vi "WindowBuild_2.vi"(7 "Init":bool, 8 "Error In":errorcluster, 11 "Fitter in":refnum<class "FitterBase.lvclass">=refnum) -> (0 "Error Out":errorcluster, 2 "Timeout":bool, 3 "Fitter out":refnum<class "FitterBase.lvclass">)   [LabVIEW 2018, in "AnalysisPlugins.lvlib" / "FitterBase.lvclass"]
uses:
  FitterBase.lvclass
  C:/projects/ICDAS/NistPluggableModules/Analysis/AnalysisPlugins/AnalysisPluginBaseClass/AnalysisPluginsBase.lvclass
  PmuAnalysisClass/PmuAnalysis.lvclass
  FGen/MemberClasses/PmuTestFunctions/PmuTestFunctions.lvclass
  AnalysisPluginBaseClass/Typedefs/SampleDataInput.ctl
  AnalysisPluginBaseClass/AnalysisPluginsBase.lvclass/AnalysisPluginsBase.ctl
  Typedefs/Wvfrm_ref.ctl
  AnalysisPluginBaseClass/Accessors/Read Window.vi
  AnalysisPluginBaseClass/Accessors/Read SensorQue.vi
  AnalysisPluginBaseClass/Accessors/Read Duration.vi
  AnalysisPluginBaseClass/Accessors/Read AnalysisTime.vi
  AnalysisPluginBaseClass/Accessors/Read SampleDataQueName.vi
  AnalysisPluginBaseClass/Accessors/Write Window.vi
  <vilib>/Utility/error.llb/Error Cluster From Error Code.vi
  <vilib>/ErrorRing/Error Ring.xnode
  AnalysisPluginBaseClass/AnalysisPluginsBase.lvclass
panel:
  out "SampleData":dbl[][](graph)
  out "Window":dbl[][](graph)
  out "T0":timestamp format="%^<%.3X\n%x>T"
  out "SensorTime":timestamp format="%^<%.3X\n%x>T"
  out "WindowTime":timestamp format="%^<%.3X\n%x>T"
  out "SampleTime":timestamp format="%^<%.3X\n%x>T"
  out "Continue":bool
  out "Valid":bool
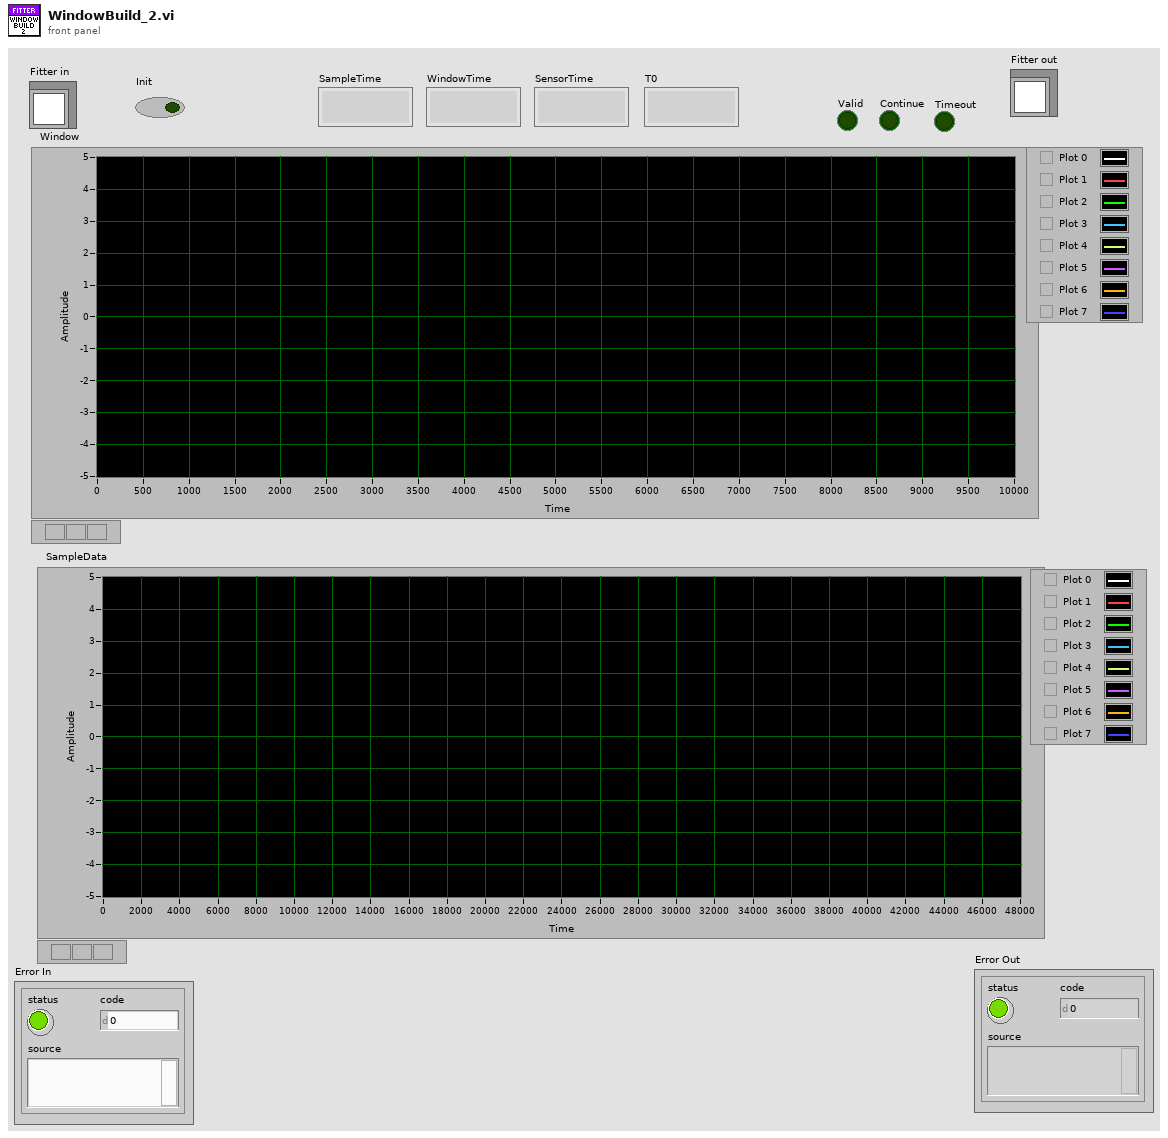
[diagram p1: front panel]
types:
  T1 = typedef "AnalysisPlugins.lvlib/AnalysisPluginsBase.lvclass/SampleDataInput.ctl" = waveform(dbl)[]
  T2 = typedef "AnalysisPlugins.lvlib/FitterBase.lvclass/Wvfrm_ref.ctl" = cluster{"t0":timestamp, "dt":dbl, "attributes":variant, "Y_ref":refnum<data-value>}
  T3 = typedef "AnalysisPlugins.lvlib/AnalysisPluginsBase.lvclass/clWindowData.ctl" = cluster{"Timestamp":ext, "Samples":dbl[][], "Window Valid":bool, "T0":ext}
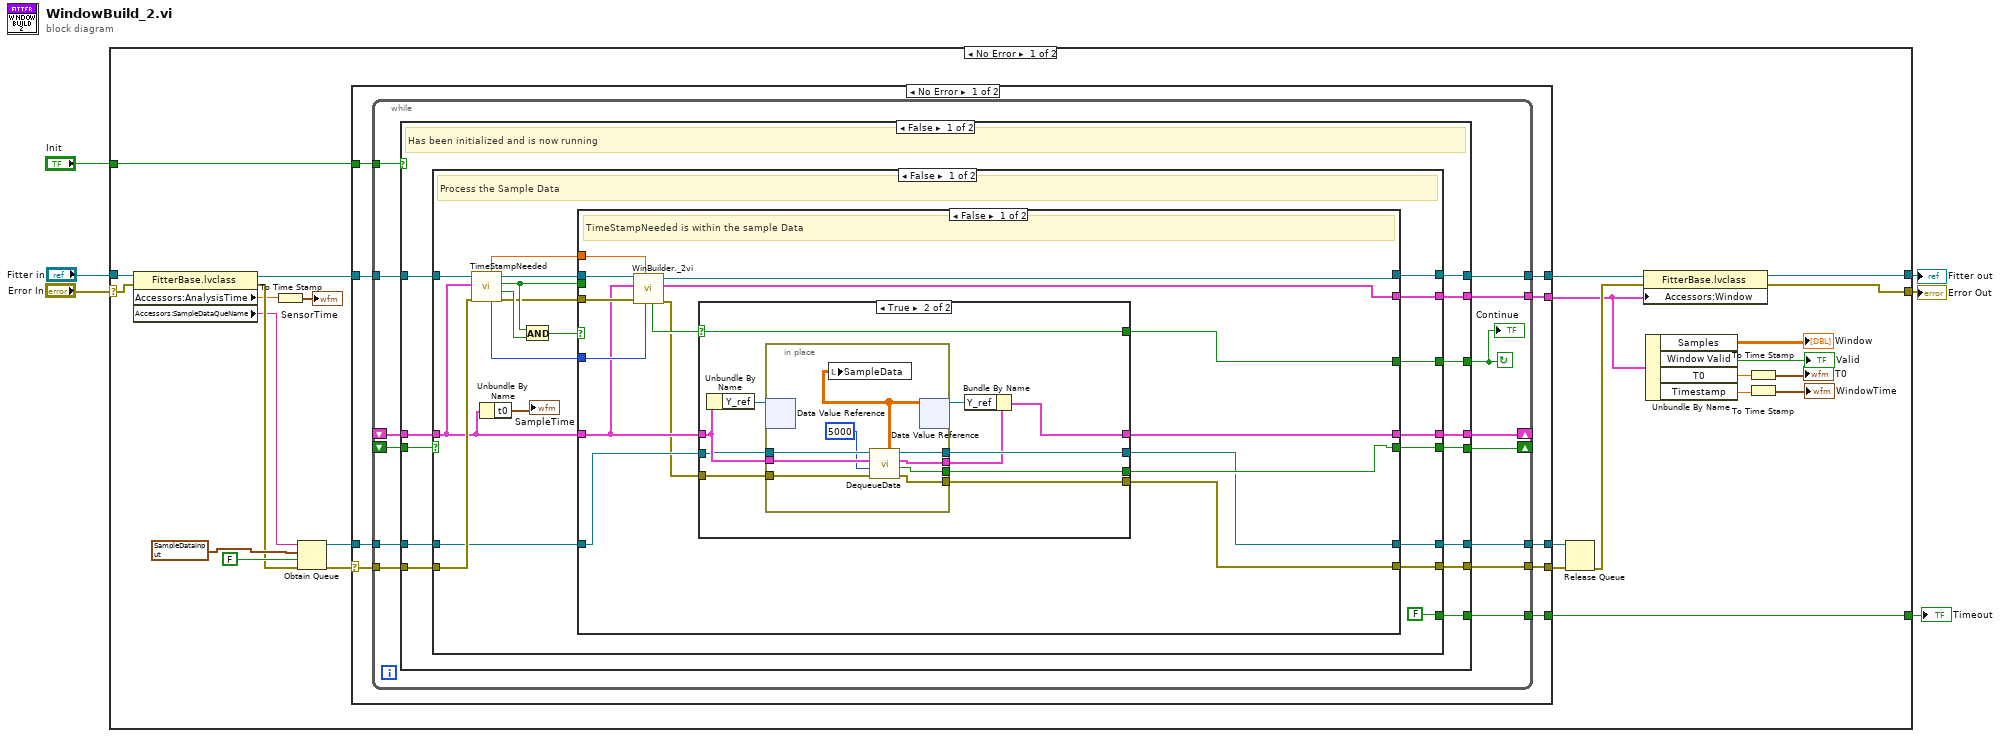
[diagram p0: block diagram]
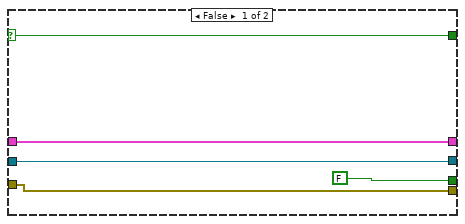
[diagram p2: hidden frame]
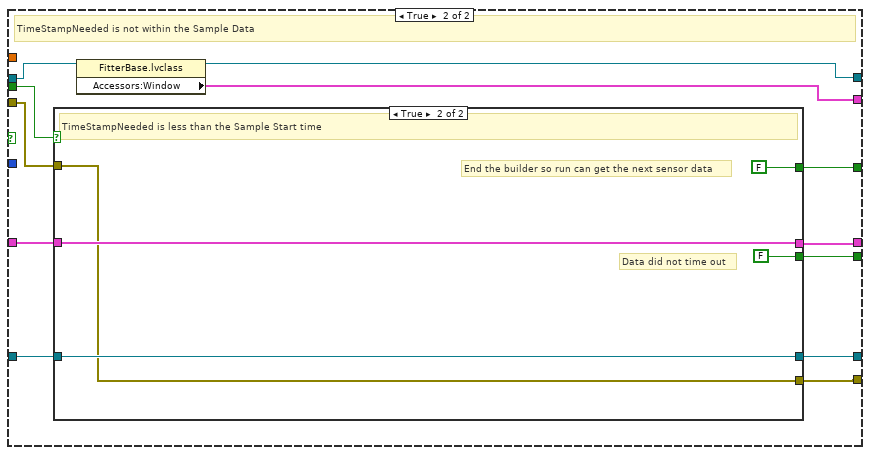
[diagram p3: hidden frame]
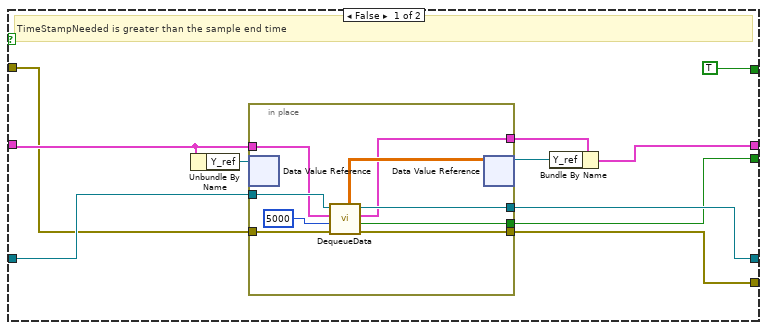
[diagram p4: hidden frame]
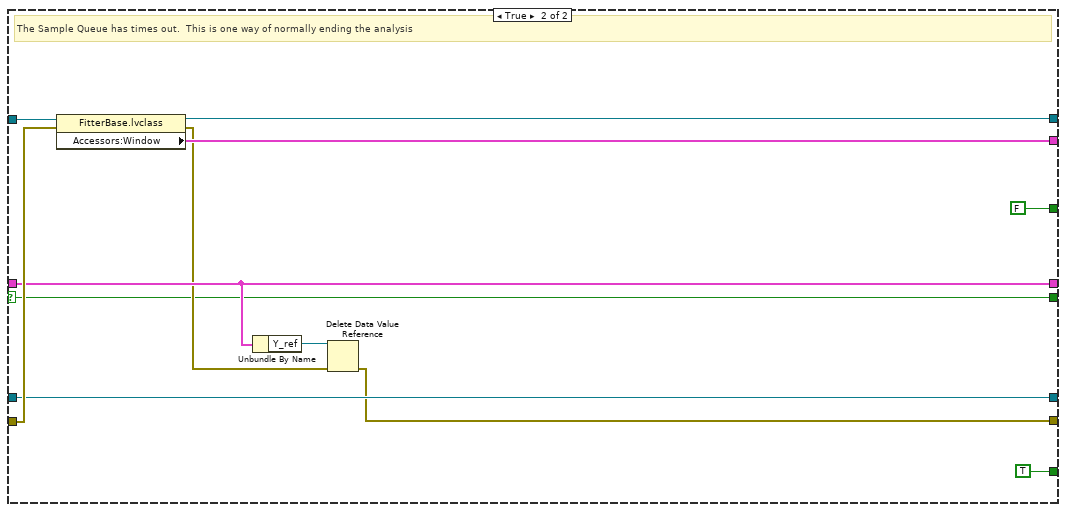
[diagram p5: hidden frame]
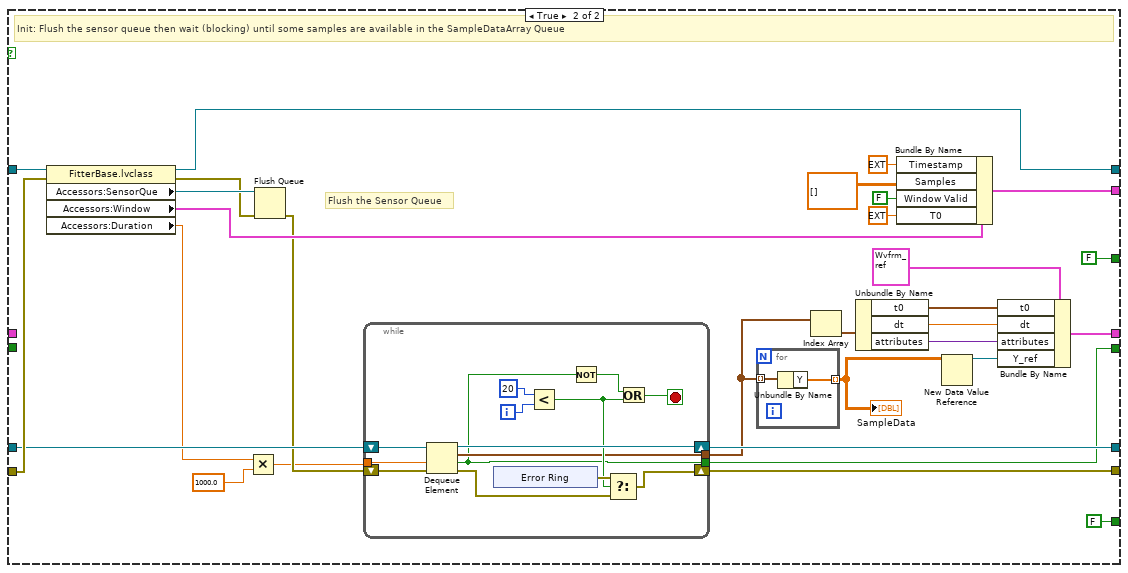
[diagram p6: hidden frame]
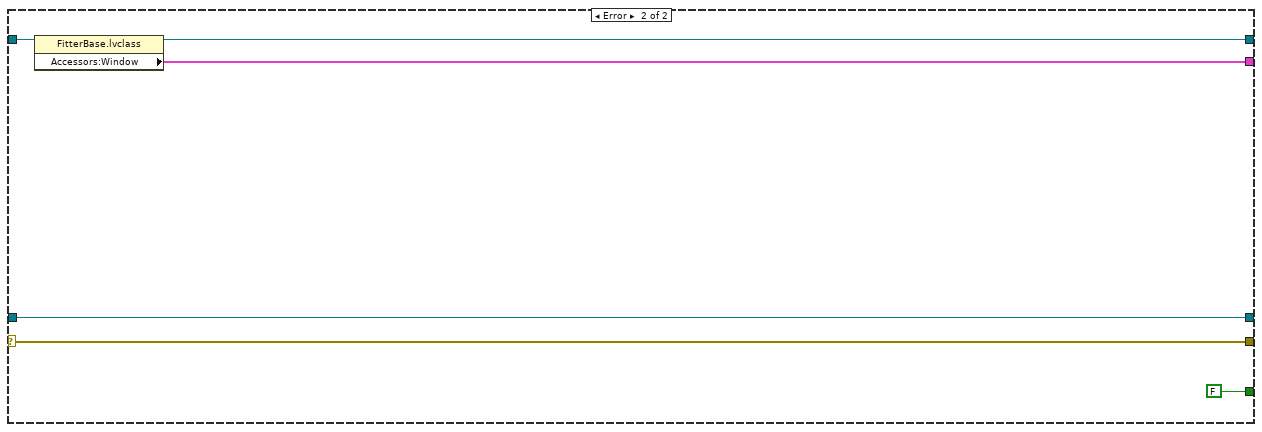
[diagram p7: hidden frame]
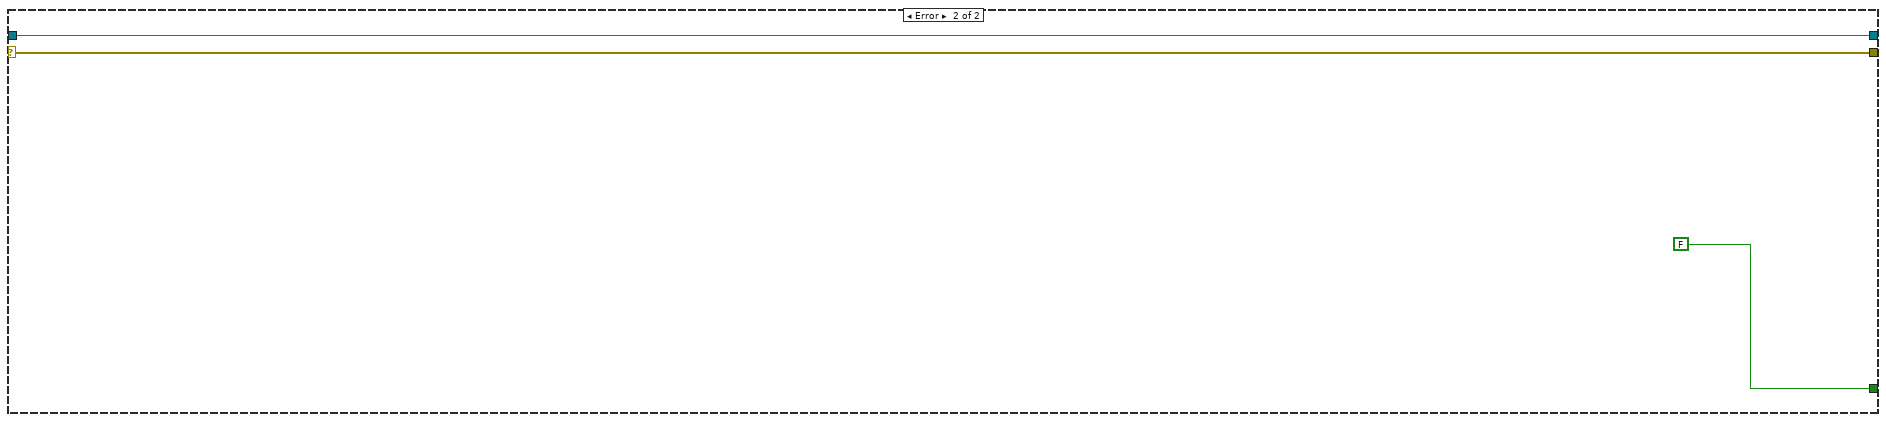
[diagram p8: hidden frame]
diagram:
  n1 = case shown="No Error" "Error In" {
    selector: "Error In" -> [w31 w235]
    tunnel: "Fitter in" -> [w32 w236]
    tunnel: [w18 w236] -> w4
    tunnel: [w17 w235] -> w3
    tunnel: [w19 FALSE] -> w2
    tunnel: "Init" -> [w20 _]
    frame No Error {
      n2 = property class="FitterBase.lvclass"(reference=w32, error in=w31) -> (reference out=w26:refnum<class "FitterBase.lvclass">, error out=w25:errorcluster, "Accessors:AnalysisTime"=w8:dbl, "Accessors:SampleDataQueName"=w9:string)
      n3 = To Time Stamp(1:w8) -> (0:→"SensorTime":timestamp)
      n4 = Obtain Queue(name (unnamed)=w9, element data type=T1 [{"t0"=timestamp(0 s since 1904-01-01), "dt"=1.0, "Y"=[]}] ("clSampleDataArray"), create if not found? (T)=FALSE, error in (no error)=w25) -> (queue out=w27:refnum<queue>, error out=w28:errorcluster)  [unwired: 1 in, 1 out]
      n5 = case shown="No Error" w28 {
        selector: w28 -> [w39 w231]
        tunnel: w27 -> [w37 w232]
        tunnel: [w33 w230] -> w22
        tunnel: w26 -> [w40 w233]
        tunnel: [w36 w232] -> w24
        tunnel: [w35 w231] -> w23
        tunnel: [w38 w229] -> w16
        tunnel: w20 -> [w41 _]
        tunnel: [w34 FALSE] -> w19
        frame No Error {
          n6 = while {
            tunnel: w41 -> [w55]
            tunnel: w40 -> [w54]
            tunnel: w39 -> [w53]
            tunnel: [w52] -> w38
            tunnel: w37 -> [w51]
            tunnel: [w50] -> w36
            tunnel: [w49] -> w35
            shift-right: [w48] -> _
            shift-left: _ -> [w43]
            shift-right: [w47] -> _
            shift-left: _ -> [w44]
            tunnel: [w46] -> w34
            tunnel: [w45] -> w33
            stop <- w42 continue-if-true
            n7 = case shown="False" w55 {
              tunnel: w54 -> [w67 w207]
              tunnel: w53 -> [w66 w206]
              tunnel: [w64 w197] -> w52
              tunnel: w51 -> [w59 w196]
              tunnel: [w58 w192] -> w50
              tunnel: [w57 w191] -> w49
              tunnel: [w62 w182] -> w48
              tunnel: [w56 w181] -> w47
              tunnel: [w60 FALSE] -> w46
              tunnel: [w61 FALSE] -> w42
              tunnel: [w65 w178] -> w45
              tunnel: w44 -> [w68 _]
              tunnel: w43 -> [w63 _]
              frame False {
                # "Has been initialized and is now running"
                n8 = case shown="False" w68 {
                  selector: w68 -> [_ w166]
                  tunnel: w67 -> [w88 w177]
                  tunnel: w66 -> [w87 w176]
                  tunnel: [w74 w175] -> w65
                  tunnel: [w73 w174] -> w64
                  tunnel: w63 -> [w70 w173]
                  tunnel: [w80 w173] -> w62
                  tunnel: [w83 FALSE] -> w61
                  tunnel: [FALSE TRUE] -> w60
                  tunnel: [w78 w168] -> w58
                  tunnel: w59 -> [w82 w168]
                  tunnel: [w79 w167] -> w57
                  tunnel: [w77 w166] -> w56
                  frame False {
                    # "Process the Sample Data"
                    n9 = call "TimeStampNeeded.vi"("Error In"=w87, "Wvfrm_ref"=w70, "Fitter In"=w88) -> ("Error Out"=w81:errorcluster, "TsnGreaterThanSampleStart"=w85:bool, "TsnLessThanSample Start Time"=w84:bool, "Fitter Out"=w76:refnum<class "FitterBase.lvclass">, "nSamplesNeeded"=w72:i32, "TimeStampNeeded"=w75:ext)  [unwired: 3 in]
                    n10 = Unbundle By Name(w70) -> ("t0"=→"SampleTime":timestamp)
                    n11 = And(x=w84, y=w85) -> (x .and. y?=w86:bool)
                    n12 = case shown="False" w86 {
                      tunnel: w84 -> [_ w140]
                      tunnel: [w95 w139] -> w83
                      tunnel: w70 -> [w97 w138]
                      tunnel: w82 -> [w94 w137]
                      tunnel: w81 -> [w102 w136]
                      tunnel: [w89 w135] -> w80
                      tunnel: [w91 w134] -> w79
                      tunnel: [w90 w133] -> w78
                      tunnel: [w92 w132] -> w77
                      tunnel: w76 -> [w103 w131]
                      tunnel: w75 -> [w101 _]
                      tunnel: [w99 w130] -> w74
                      tunnel: [w98 w129] -> w73
                      tunnel: w72 -> [w100 _]
                      frame False {
                        # "TimeStampNeeded is within the sample Data"
                        n13 = call "WinBuilder._2vi.vi"("nSampleNeeded"=w100, "TimeStampNeeded"=w101, "Error In"=w102, "Wvfrm_ref"=w97, "Fitter In"=w103) -> ("Error Out"=w93:errorcluster, "Window"=w98:T3, "Fitter Out"=w99:refnum<class "FitterBase.lvclass">, "Continue"=w96:bool)  [unwired: 2 in, 1 out]
                        n14 = case shown="True" w96 {
                          selector: w96 -> [w105 w113]
                          tunnel: w94 -> [w108 w117]
                          tunnel: w97 -> [w107 w119]
                          tunnel: w93 -> [w106 w116]
                          tunnel: [w108 w115] -> w90
                          tunnel: [w107 w110] -> w89
                          tunnel: [w106 w114] -> w91
                          tunnel: [w105 w113] -> w95
                          tunnel: [FALSE w112] -> w92
                          frame False {
                          }
                          frame True {
                            n15 = Unbundle By Name(w119) -> ("Y_ref"=w118:refnum<data-value>)
                            n16 = in-place {
                              in-place-border: w119 -> [w127]
                              in-place-border: w117 -> [w128]
                              in-place-border: w116 -> [w125]
                              in-place-border: [w124] -> w115
                              in-place-border: [w123] -> w111
                              in-place-border: [w122] -> w112
                              in-place-border: [w121] -> w114
                              n17 = in-place-dvr #1(w118) -> ()  [unwired: 2 out]
                              n18 = call "DequeueData.vi"("error in (no error)"=w125, "timeout in ms (-1)"=5000, "DataIn"=w127, "queue in"=w128) -> ("error out"=w121:errorcluster, "timed out?"=w122:bool, "Data Out"=w123:T2, "queue out"=w124:refnum<queue>, "Y"=w120:dbl[][])  [unwired: 3 in]
                              n19 = local write "SampleData"(w120) -> ()
                              n20 = in-place-dvr #1(w120) -> (w109:refnum<data-value>)  [unwired: 1 out]
                            }
                            n21 = Bundle By Name(cluster=w111, "Y_ref"=w109) -> (w110:T2)
                          }
                        }
                      }
                      frame True {
                        # "TimeStampNeeded is not within the Sample Data"
                        n22 = case shown="True" w140 {
                          tunnel: [TRUE FALSE] -> w139
                          tunnel: w138 -> [w147 w164]
                          tunnel: w137 -> [w146 w162]
                          tunnel: w136 -> [w145 w161]
                          tunnel: [w144 w164] -> w135
                          tunnel: [w143 w161] -> w134
                          tunnel: [w142 w162] -> w133
                          tunnel: [w141 FALSE] -> w132
                          frame False {
                            # "TimeStampNeeded is greater than the sample end time"
                            n23 = Unbundle By Name(w147) -> ("Y_ref"=w148:refnum<data-value>)
                            n24 = in-place {
                              in-place-border: w145 -> [w160]
                              in-place-border: w146 -> [w158]
                              in-place-border: w147 -> [w157]
                              in-place-border: [w156] -> w142
                              in-place-border: [w155] -> w143
                              in-place-border: [w154] -> w141
                              in-place-border: [w152] -> w149
                              n25 = in-place-dvr #2(w148) -> ()  [unwired: 2 out]
                              n26 = call "DequeueData.vi"("error in (no error)"=w160, "timeout in ms (-1)"=5000, "DataIn"=w157, "queue in"=w158) -> ("error out"=w155:errorcluster, "timed out?"=w154:bool, "Data Out"=w152:T2, "queue out"=w156:refnum<queue>, "Y"=w153:dbl[][])  [unwired: 3 in]
                              n27 = in-place-dvr #2(w153) -> (w150:refnum<data-value>)  [unwired: 1 out]
                            }
                            n28 = Bundle By Name(cluster=w149, "Y_ref"=w150) -> (w144:T2)
                          }
                          frame True {
                            # "Data did not time out"
                            # "End the builder so run can get the next sensor data"
                            # "TimeStampNeeded is less than the Sample Start time"
                          }
                        }
                        n29 = property class="FitterBase.lvclass"(reference=w131) -> (reference out=w130:refnum<class "FitterBase.lvclass">, "Accessors:Window"=w129:T3)  [unwired: 1 in, 1 out]
                      }
                    }
                  }
                  frame True {
                    # "The Sample Queue has times out.  This is one way of normally ending the analysis"
                    n30 = property class="FitterBase.lvclass"(reference=w177, error in=w176) -> (reference out=w175:refnum<class "FitterBase.lvclass">, error out=w171:errorcluster, "Accessors:Window"=w174:T3)
                    n31 = Unbundle By Name(w173) -> ("Y_ref"=w172:refnum<data-value>)
                    n32 = Delete Data Value Reference(data value reference=w172, error in=w171) -> (error out=w167:errorcluster)  [unwired: 1 out]
                  }
                }
              }
              frame True {
                # "Flush the Sensor Queue"
                # "Init: Flush the sensor queue then wait (blocking) until some samples are available in the SampleDataArray Queue"
                n33 = property class="FitterBase.lvclass"(reference=w207, error in=w206) -> (reference out=w178:refnum<class "FitterBase.lvclass">, error out=w203:errorcluster, "Accessors:SensorQue"=w204:refnum<queue>, "Accessors:Window"=w202:T3, "Accessors:Duration"=w194:dbl)
                n34 = Multiply(x=w194, y=1000.0) -> (x*y=w193:dbl)
                n35 = Flush Queue(queue=w204, error in (no error)=w203) -> (error out=w195:errorcluster)  [unwired: 2 out]
                n36 = while {
                  shift-right: [w218] -> w192
                  shift-left: w196 -> [w223]
                  shift-right: [w219] -> w191
                  shift-left: w195 -> [w222]
                  tunnel: w193 -> [w213]
                  tunnel: [w211] -> w184
                  tunnel: [w210] -> w181
                  i -> [w215]
                  stop <- w212 stop-if-true
                  n37 = Dequeue Element(queue=w223, timeout in ms (-1)=w213, error in (no error)=w222) -> (queue out=w218:refnum<queue>, element=w211:T1, timed out?=w210:bool, error out=w220:errorcluster)
                  n38 = xnode "Error Ring"() -> ("error out"=w221:errorcluster)
                  n39 = Less?(x=20 ("timeout in ms (-1)"), y=w215) -> (x < y?=w214:bool)
                  n40 = Not(x=w210) -> (.not. x?=w217:bool)
                  n41 = Select(t=w221, s=w214, f=w220) -> (s? t:f=w219:errorcluster)
                  n42 = Or(x=w217, y=w214) -> (x .or. y?=w212:bool)
                }
                n43 = for {
                  tunnel: w184 -> [w209] mode=indexing
                  tunnel: [w208] -> w183 mode=indexing
                  n44 = Unbundle By Name(w209) -> ("Y"=w208:dbl[])
                }
                "SampleData" <- w183
                n45 = Index Array(array=w184) -> (element=w190:waveform(dbl))  [unwired: 1 in]
                n46 = Unbundle By Name(w190) -> ("t0"=w188:timestamp, "dt"=w187:dbl, "attributes"=w186:variant)
                n47 = Bundle By Name(cluster=w202, "Timestamp"=ext 0.0, "Samples"=dbl[][] [], "Window Valid"=FALSE, "T0"=ext -1.0) -> (w197:T3)
                n48 = New Data Value Reference(data value=w183) -> (data value reference=w185:refnum<data-value>)  [unwired: 1 in, 1 out]
                n49 = Bundle By Name(cluster=T2 {"t0"=timestamp(0 s since 1904-01-01), "dt"=1.0, "attributes"=variant, "Y_ref"=refnum} ("Wvfrm_ref"), "t0"=w188, "dt"=w187, "attributes"=w186, "Y_ref"=w185) -> (w182:T2)
              }
            }
            "Continue" <- w42
          }
        }
        frame Error {
          n50 = property class="FitterBase.lvclass"(reference=w233) -> (reference out=w230:refnum<class "FitterBase.lvclass">, "Accessors:Window"=w229:T3)  [unwired: 1 in, 1 out]
        }
      }
      n51 = Release Queue(queue=w24, error in (no error)=w23) -> (error out=w21:errorcluster)  [unwired: 1 in, 2 out]
      n52 = property class="FitterBase.lvclass"(reference=w22, error in=w21, "Accessors:Window"=w16) -> (reference out=w18:refnum<class "FitterBase.lvclass">, error out=w17:errorcluster)
      n53 = Unbundle By Name(w16) -> ("Samples"=→"Window":dbl[][], "Window Valid"=→"Valid":bool, "T0"=w13:ext, "Timestamp"=w11:ext)
      n54 = To Time Stamp(1:w13) -> (0:→"T0":timestamp)
      n55 = To Time Stamp(1:w11) -> (0:→"WindowTime":timestamp)
    }
    frame Error {
    }
  }
  "Fitter out" <- w4
  "Timeout" <- w2
  "Error Out" <- w3
